vi "IT8800-Query Operation.vi"(8 "error in":errorcluster, 11 "IT8800 Setting In In":T1={"VISA Resource Name"="", "Baud Rate"=19200, "Stop Bits"=20, "Wait For Read(ms)"=0, "Interface Type"=enum."VXI", "Limits"=[]} {"Stop Bits" items=["1.0"=10, "2.0"=20]; "Baud Rate" items=["2400"=2400, "4800"=4800, "9600"=9600, "19200"=19200]}) -> (0 "error out":errorcluster, 2 "Operation Mode":T2, 3 "IT8800 Setting In Out":T1={"VISA Resource Name"="", "Baud Rate"=19200, "Stop Bits"=20, "Wait For Read(ms)"=0, "Interface Type"=enum."VXI", "Limits"=[]} {"Stop Bits" items=["1.0"=10, "2.0"=20]; "Baud Rate" items=["2400"=2400, "4800"=4800, "9600"=9600, "19200"=19200]})   [LabVIEW 2018]
uses:
  Data Def/IT8800-Operation Mode.ctl
  Data Def/IT8800-Setting.ctl
panel:
  out "Response":string
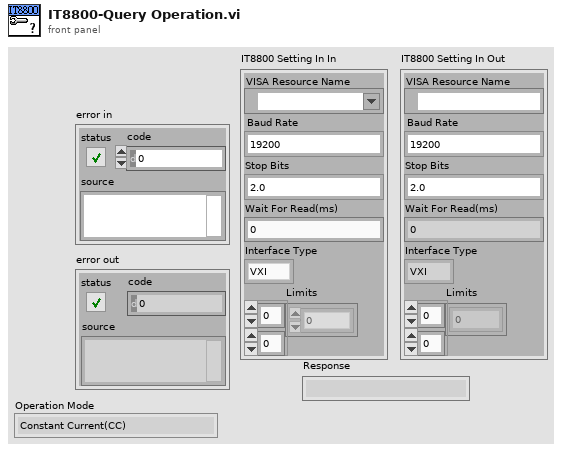
[diagram p1: front panel]
types:
  T1 = typedef "IT8800-Setting.ctl" = cluster{"VISA Resource Name":refnum<visa-resource-name>, "Baud Rate":u32, "Stop Bits":u16, "Wait For Read(ms)":u32, "Interface Type":enum16{"Unknow", "GPIB", "VXI", "GPIB-VXI", "Serial", "PXI", "TCPIP", "USB", "FireWire"}, "Limits":dbl[][]}
  T2 = typedef "IT8800-Operation Mode.ctl" = enum16{"Constant Current(CC)", "Constant Voltage(CV)", "Constant Power(CP)", "Constant Resistance(CR)"}
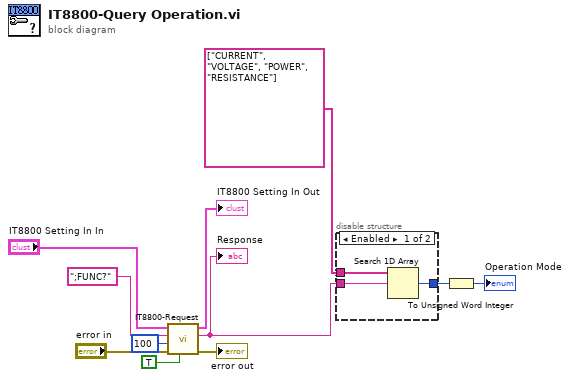
[diagram p0: block diagram]
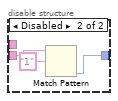
[diagram p2: hidden frame]
diagram:
  n1 = call "IT8800-Request.vi"("Response?"=TRUE, "error in"="error in", "byte count"=u32 100, "Command"=";FUNC?", "IT8800 Setting In In"="IT8800 Setting In In") -> ("error out"=→"error out":errorcluster, "Response"=w8:string, "IT8800 Setting In Out"=→"IT8800 Setting In Out":T1)  [unwired: 4 in]
  "Response" <- w8
  n2 = disable-structure shown="Enabled" {
    disable-tunnel: w8 -> [w14 w17]
    disable-tunnel: string[] ["CURRENT", "VOLTAGE", "POWER", "RESISTANCE"] -> [w13 _]
    disable-tunnel: [w12 w15] -> w6
    frame Enabled {
      n3 = Search 1D Array(1D array=w13, element=w14) -> (index of element=w12:i32)  [unwired: 1 in]
    }
    frame Disabled {
      n4 = Match Pattern(string=w17, regular expression="1") -> (offset past match=w15:i32)  [unwired: 1 in, 3 out]
    }
  }
  n5 = To Unsigned Word Integer(number=w6) -> (unsigned 16bit integer=→"Operation Mode":u16)
